vi "Instrument Create and Download Script.vi"(0 "RFSG handle":refnum<k15>, 5 "PAEN Timing in":T2={"tRF (s)"=0.0, "Duty Cycle"=50.0, "t1 (s)"=5e-07, "t2 (s)"=5e-07, "t3 (s)"=0.0, "Period (s)"=0.0, "WLAN PFI Mode"=enum."Static"} {"Period (s)" format="%#_5p"; "t3 (s)" min=0.0 step=0.01 format="%#_5p"; "t2 (s)" min=0.0 max=0.1 step=0.01 format="%#_3p"; "t1 (s)" min=0.0 max=0.1 step=0.01 format="%#_3p"; "Duty Cycle" min=1.0 max=100.0 step=1.0 format="%#_2d%%"; "tRF (s)" min=0.0 step=0.01 format="%#_5p"}, 7 "Waveform":T1={"Waveform"={"x0"=0.0, "dx"=0.0, "y"=[]}, "Idle Duration Present"=0, "PAPR (dB)"=0.0, "Waveform Name"="Wfm", "Burst Start Locations"=[], "Burst Stop Locations"=[], "Script Name"="Wfm", "Signal Bandwidth (Hz)"=0.0, "Burst Length (s)"=0.0, "LO Frequency Offset (Hz)"=0.0} {"Burst Length (s)" format="%#_6p"; "Signal Bandwidth (Hz)" format="%#_6p"; "PAPR (dB)" format="%.2f"; "Idle Duration Present" items=["False", "True"]; "Waveform"."y" format="%.2f"; "Waveform"."dx" format="%^.2e"; "Waveform"."x0" format="%^.2e"}, 11 "error in":errorcluster) -> (4 "RFSG handle out":refnum<k15>, 6 "PAEN Timing out":T2={"tRF (s)"=0.0, "Duty Cycle"=50.0, "t1 (s)"=5e-07, "t2 (s)"=5e-07, "t3 (s)"=0.0, "Period (s)"=0.0, "WLAN PFI Mode"=enum."Static"} {"Period (s)" format="%#_5p"; "t3 (s)" min=0.0 step=0.01 format="%#_5p"; "t2 (s)" min=0.0 max=0.1 step=0.01 format="%#_3p"; "t1 (s)" min=0.0 max=0.1 step=0.01 format="%#_3p"; "Duty Cycle" min=1.0 max=100.0 step=1.0 format="%#_2d%%"; "tRF (s)" min=0.0 step=0.01 format="%#_5p"}, 15 "error out":errorcluster)   [LabVIEW 2018, in "SG.lvlib"]
uses:
  SG.lvlib
  Typedefs/PAEN Timing.ctl
  Typedefs/Waveform.ctl
  <instrlib>/niRFSG/niRFSG.llb/niRFSG Signal Names.ctl
  <instrlib>/niRFSG/niRFSG.llb/niRFSG Signal Identifiers.ctl
  <instrlib>/niRFSG/niRFSG.llb/niRFSG Exported Signal Destinations.ctl
  <instrlib>/niRFSGPlayback/niRFSGPlayback Set Script to Generate (1 RFSG).vi
  Utilities/RDLUtilities.lvlib
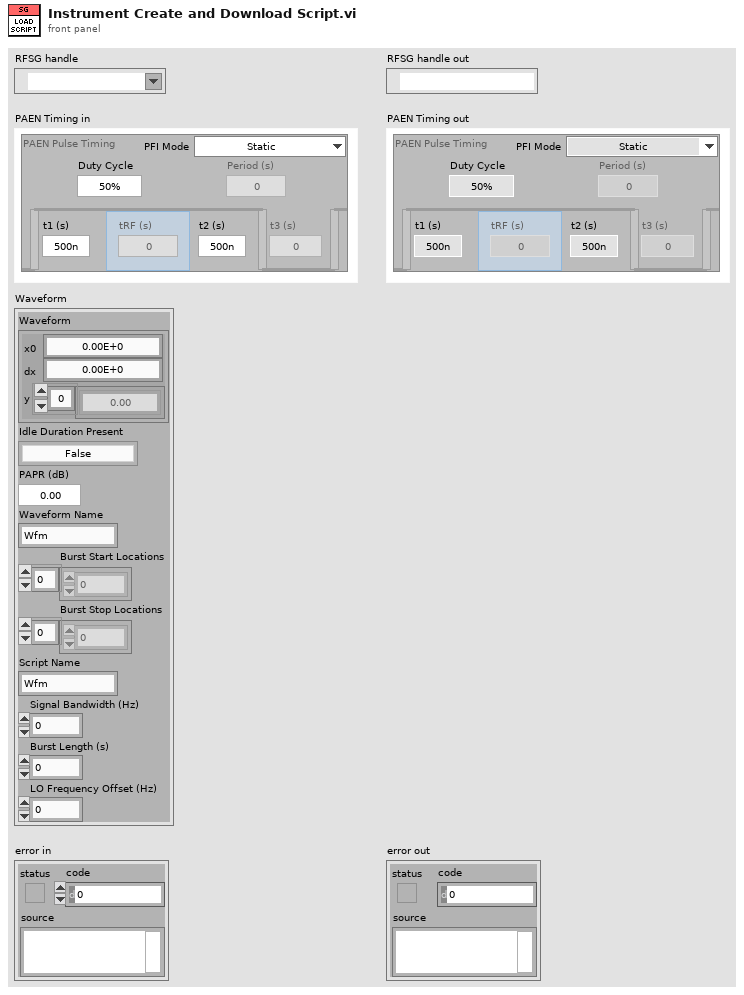
[diagram p1: front panel]
types:
  T1 = typedef "SG.lvlib/Waveform.ctl" = cluster{"Waveform":cluster{"x0":dbl, "dx":dbl, "y":csg[]}, "Idle Duration Present":i32, "PAPR (dB)":dbl, "Waveform Name":string, "Burst Start Locations":i32[], "Burst Stop Locations":i32[], "Script Name":string, "Signal Bandwidth (Hz)":dbl, "Burst Length (s)":dbl, "LO Frequency Offset (Hz)":dbl}
  T2 = typedef "SG.lvlib/PAEN Timing.ctl" = cluster{"tRF (s)":dbl, "Duty Cycle":dbl, "t1 (s)":dbl, "t2 (s)":dbl, "t3 (s)":dbl, "Period (s)":dbl, "WLAN PFI Mode":enum16{"Static", "Dynamic"}}
  T3 = typedef "niRFSG Exported Signal Destinations.ctl" = string
  T4 = typedef "niRFSG Signal Identifiers.ctl" = string
  T5 = typedef "niRFSG Signal Names.ctl" = i32
  T6 = cluster{"tRF (s)":dbl, "Duty Cycle":dbl, "t1 (s)":dbl, "t2 (s)":dbl, "t3 (s)":dbl, "Period (s)":dbl, "WLAN PFI Mode":dbl}
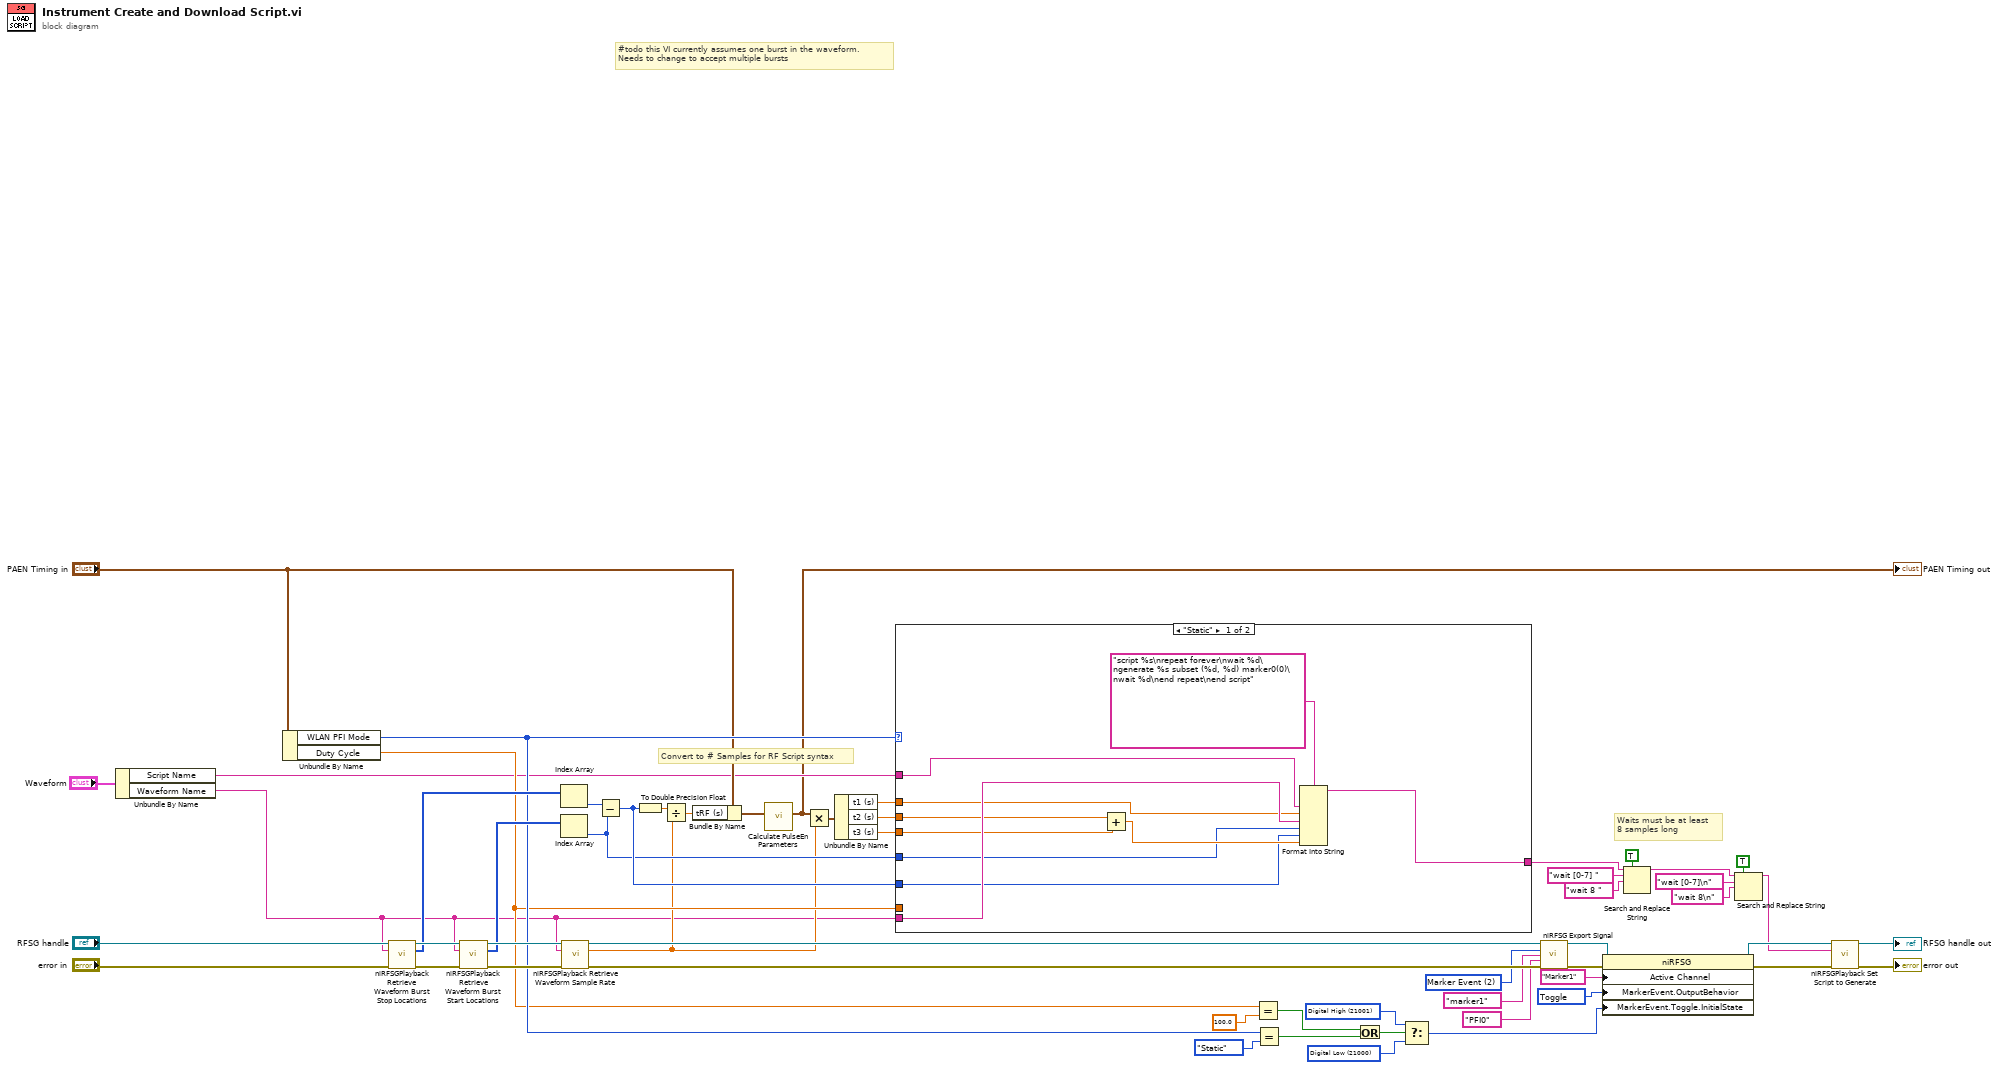
[diagram p0: block diagram]
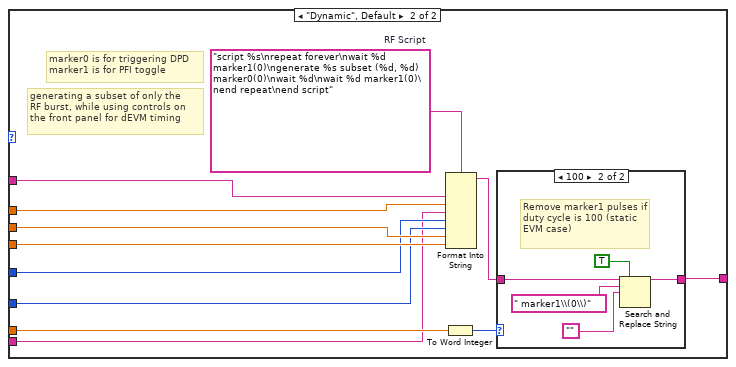
[diagram p2: hidden frame]
diagram:
  w24 = 21000 items=["Digital Low"=21000, "Digital High"=21001] ("Events:Marker:Toggle:Initial State")
  w23 = 21001 items=["Digital Low"=21000, "Digital High"=21001] ("Events:Marker:Toggle:Initial State")
  w30 = T5 2 items=["Start Trigger", "Script Trigger", "Marker Event", "Ref Clock", "Started Event", "Done Event", "Configuration List Step Trigger", "Configuration Settled Event"] ("signal")
  w29 = 23001 items=["Pulse"=23000, "Toggle"=23001] ("Events:Marker:Output Behavior")
  # "Convert to # Samples for RF Script syntax"
  # "Waits must be at least \n8 samples long"
  # "#todo this VI currently assumes one burst in the waveform.\nNeeds to change to accept multiple bursts"
  n1 = Unbundle By Name("Waveform") -> ("Script Name"=w5:string, "Waveform Name"=w4:string)
  n2 = Unbundle By Name("PAEN Timing in") -> ("WLAN PFI Mode"=w12:enum16{"Static", "Dynamic"}, "Duty Cycle"=w11:dbl)
  n3 = call <instrlib>:"niRFSGPlayback Retrieve Waveform Burst Stop Locations.vi"("instrument handle in"="RFSG handle", "waveform name"=w4, "error in"="error in") -> ("instrument handle out"=w14:refnum<k15>, "burst stop locations"=w13:i32[], "error out"=w50:errorcluster)  [unwired: 10 in]
  n4 = call <instrlib>:"niRFSGPlayback Retrieve Waveform Burst Start Locations.vi"("instrument handle in"=w14, "waveform name"=w4, "error in"=w50) -> ("instrument handle out"=w17:refnum<k15>, "burst start locations"=w16:i32[], "error out"=w51:errorcluster)  [unwired: 10 in]
  n5 = Index Array(array=w13) -> (element=w42:i32)  [unwired: 1 in]
  n6 = Index Array(array=w16) -> (element=w8:i32)  [unwired: 1 in]
  n7 = call <instrlib>:"niRFSGPlayback Retrieve Waveform Sample Rate.vi"("instrument handle in"=w17, "waveform name"=w4, "error in"=w51) -> ("instrument handle out"=w27:refnum<k15>, "sample rate"=w7:dbl, "error out"=w53:errorcluster)  [unwired: 10 in]
  n8 = Subtract(x=w42, y=w8) -> (x-y=w35:i32)
  n9 = To Double Precision Float(number=w35) -> (double precision float=w41:dbl)
  n10 = Divide(x=w41, y=w7) -> (x/y=w40:dbl)
  n11 = Bundle By Name(cluster="PAEN Timing in", "tRF (s)"=w40) -> (w18:T2)
  n12 = call "Calculate PulseEn Parameters.vi"("PAEN Timing In"=w18) -> ("PAEN Timing Out"=w1:T2)  [unwired: 10 in]
  "PAEN Timing out" <- w1
  n13 = Multiply(x=w1, y=w7) -> (x*y=w39:T6)
  n14 = Unbundle By Name(w39) -> ("t1 (s)"=w36:dbl, "t2 (s)"=w37:dbl, "t3 (s)"=w38:dbl)
  n15 = case shown="\"Static\"" w12 {
    tunnel: w11 -> [_ w76]
    tunnel: w38 -> [w57 w75]
    tunnel: w37 -> [w62 w74]
    tunnel: w36 -> [w63 w73]
    tunnel: w5 -> [w65 w72]
    tunnel: w8 -> [w60 w71]
    tunnel: w35 -> [w61 w70]
    tunnel: w4 -> [w64 w69]
    tunnel: [w59 w67] -> w33
    frame "Static" {
      n16 = Add(x=w62, y=w57) -> (x+y=w66:dbl)
      n17 = Format Into String(format string="script %s\nrepeat forever\nwait %d\ngenerate %s subset (%d, %d) marker0(0)\nwait %d\nend repeat\nend script", w65, w63, w64, w60, w61, w66) -> (resulting string=w59:string)  [unwired: 2 in, 1 out]
    }
    frame "Dynamic", Default {
      w77 = "script %s\nrepeat forever\nwait %d marker1(0)\ngenerate %s subset (%d, %d) marker0(0)\nwait %d\nwait %d marker1(0)\nend repeat\nend script"  # RF Script
      # "generating a subset of only the\nRF burst, while using controls on\nthe front panel for dEVM timing"
      # "marker0 is for triggering DPD\nmarker1 is for PFI toggle"
      n18 = To Word Integer(number=w76) -> (16bit integer=w78:i16)
      n19 = Format Into String(format string=w77, w72, w73, w69, w71, w70, w74, w75) -> (resulting string=w68:string)  [unwired: 2 in, 1 out]
      n20 = case shown="100" w78 {
        tunnel: w68 -> [w79 w81]
        tunnel: [w79 w80] -> w67
        frame Default {
        }
        frame 100 {
          # "Remove marker1 pulses if duty cycle is 100 (static EVM case)"
          n21 = Search and Replace String(replace all?=TRUE ("replace all? (F)"), input string=w81, search string=" marker1\\(0\\)", replace string="" ("replace string (\"\")")) -> (result string=w80:string)  [unwired: 4 in, 3 out]
        }
      }
    }
  }
  n22 = Equal?(x=w11, y=100.0) -> (x = y?=w19:bool)
  n23 = Equal?(x=w12, y=enum16{"Static", "Dynamic"}."Static" ("PAEN Timing.WLAN PFI Mode")) -> (x = y?=w25:bool)
  n24 = Or(x=w19, y=w25) -> (x .or. y?=w20:bool)
  n25 = Select(t=w23, s=w20, f=w24) -> (s? t:f=w22:i32)
  n26 = call <instrlib>:"niRFSG Export Signal.vi"("instrument handle"=w27, "signal"=w30, "signal identifier"=T4 "marker1", "output terminal"=T3 "PFI0", "error in"=w53) -> ("instrument handle out"=w9:refnum<k15>, "error out"=w54:errorcluster)  [unwired: 9 in]
  n27 = property class="niRFSG"(reference=w9, error in=w54, "Active Channel"="Marker1", "MarkerEvent.OutputBehavior"=w29, "MarkerEvent.Toggle.InitialState"=w22) -> (reference out=w3:refnum<k15>, error out=w52:errorcluster)
  n28 = Search and Replace String(replace all?=TRUE ("replace all? (F)"), input string=w33, search string="wait [0-7] ", replace string="wait 8 " ("replace string (\"\")")) -> (result string=w49:string)  [unwired: 4 in, 3 out]
  n29 = Search and Replace String(replace all?=TRUE ("replace all? (F)"), input string=w49, search string="wait [0-7]\n", replace string="wait 8\n" ("replace string (\"\")")) -> (result string=w2:string)  [unwired: 4 in, 3 out]
  n30 = call-poly <instrlib>:"niRFSGPlayback Set Script to Generate.vi"("instrument handle in"=w3, "script text"=w2, "error in"=w52) -> ("instrument handle out"=→"RFSG handle out":refnum<k15>, "error out"=→"error out":errorcluster)  [unwired: 11 in]
